vi "energy scan.vi"() -> ()   [LabVIEW 2013]
uses:
  <vilib>/Utility/file.llb/Write To Spreadsheet File (I64).vi
panel:
  in  "encoder enable":bool
  in  "2nd motor enable":bool=TRUE
  out "status":string="motion complete"
  in  "filename":string="cu_foil_Kalpha_01.txt"
  in  "file path":path=path "C:/Users/seidler/Documents/lab XANES software/lab XES data/Joe/Si_111_2013_12_09"
  out "step number":i32=399
  out "detector encoder":string="-189735\r"
  out "source encoder":string="-151316\r"
  in  "detector motor":u16(ring)=5 items=["theta"=1, "chi"=2, "rho"=3, "source"=4, "detector"=5, "sample"=6]
  in  "source motor":u16(ring)=4 items=["theta"=1, "chi"=2, "rho"=3, "source"=4, "detector"=5, "sample"=6]
  out "XY Graph":cluster{i32[], i32[]}(graph)={[0, 1, 2, 3, 4, 5, 6, 7, 8, 9, 10, 11, 12, 13, 14, 15, 16, 17, 18, 19, 20, 21, 22, 23, 24, 25, 26, 27, 28, 29, 30, 31, 32, 33, 34, 35, 36, 37, 38, 39, 40, 41, 42, 43, 44, 45, 46, 47, 48, 49, 50, 51, 52, 53, 54, 55, 56, 57, 58, 59, 60, 61, 62, 63, 64, 65, 66, 67, 68, 69, 70, 71, 72, 73, 74, 75, 76, 77, 78, 79, 80, 81, 82, 83, 84, 85, 86, 87, 88, 89, 90, 91, 92, 93, 94, 95, 96, 97, 98, 99, 100, 101, 102, 103, 104, 105, 106, 107, 108, 109, 110, 111, 112, 113, 114, 115, 116, 117, 118, 119, 120, 121, 122, 123, 124, 125, 126, 127, 128, 129, 130, 131, 132, 133, 134, 135, 136, 137, 138, 139, 140, 141, 142, 143, 144, 145, 146, 147, 148, 149, 150, 151, 152, 153, 154, 155, 156, 157, 158, 159, 160, 161, 162, 163, 164, 165, 166, 167, 168, 169, 170, 171, 172, 173, 174, 175, 176, 177, 178, 179, 180, 181, 182, 183, 184, 185, 186, 187, 188, 189, 190, 191, 192, 193, 194, 195, 196, 197, 198, 199, 200, 201, 202, 203, 204, 205, 206, 207, 208, 209, 210, 211, 212, 213, 214, 215, 216, 217, 218, 219, 220, 221, 222, 223, 224, 225, 226, 227, 228, 229, 230, 231, 232, 233, 234, 235, 236, 237, 238, 239, 240, 241, 242, 243, 244, 245, 246, 247, 248, 249, 250, 251, 252, 253, 254, 255, 256, 257, 258, 259, 260, 261, 262, 263, 264, 265, 266, 267, 268, 269, 270, 271, 272, 273, 274, 275, 276, 277, 278, 279, 280, 281, 282, 283, 284, 285, 286, 287, 288, 289, 290, 291, 292, 293, 294, 295, 296, 297, 298, 299, 300, 301, 302, 303, 304, 305, 306, 307, 308, 309, 310, 311, 312, 313, 314, 315, 316, 317, 318, 319, 320, 321, 322, 323, 324, 325, 326, 327, 328, 329, 330, 331, 332, 333, 334, 335, 336, 337, 338, 339, 340, 341, 342, 343, 344, 345, 346, 347, 348, 349, 350, 351, 352, 353, 354, 355, 356, 357, 358, 359, 360, 361, 362, 363, 364, 365, 366, 367, 368, 369, 370, 371, 372, 373, 374, 375, 376, 377, 378, 379, 380, 381, 382, 383, 384, 385, 386, 387, 388, 389, 390, 391, 392, 393, 394, 395, 396, 397, 398, 399], [20, 23, 14, 17, 19, 21, 27, 19, 23, 16, 20, 22, 21, 26, 21, 24, 21, 18, 21, 19, 27, 23, 25, 22, 24, 16, 18, 25, 21, 25, 23, 25, 27, 19, 22, 24, 33, 27, 26, 34, 32, 24, 23, 26, 35, 29, 31, 28, 35, 30, 26, 41, 38, 38, 30, 30, 36, 47, 43, 44, 45, 42, 48, 49, 47, 49, 31, 53, 49, 50, 52, 51, 57, 66, 63, 64, 68, 75, 68, 89, 74, 64, 104, 113, 94, 106, 98, 158, 133, 141, 186, 184, 192, 200, 225, 279, 242, 314, 312, 398, 411, 502, 542, 520, 736, 787, 859, 960, 1045, 1179, 1285, 1496, 1544, 1613, 1606, 1665, 1557, 1592, 1469, 1286, 1135, 1030, 895, 831, 689, 643, 516, 428, 422, 349, 296, 271, 241, 229, 211, 211, 147, 172, 154, 140, 158, 137, 126, 117, 129, 112, 104, 122, 113, 112, 92, 79, 103, 83, 81, 100, 110, 97, 101, 103, 101, 84, 85, 119, 114, 121, 136, 139, 153, 159, 163, 158, 167, 186, 225, 202, 228, 236, 267, 293, 311, 352, 408, 472, 504, 589, 643, 722, 784, 911, 978, 1183, 1299, 1571, 1750, 2049, 2227, 2431, 2892, 3020, 3211, 3089, 3132, 3048, 2655, 2402, 2016, 1808, 1581, 1335, 1056, 877, 736, 607, 591, 492, 403, 363, 344, 264, 239, 269, 221, 218, 184, 173, 149, 143, 133, 124, 115, 107, 105, 94, 80, 84, 74, 78, 72, 64, 63, 56, 51, 42, 56, 48, 42, 45, 45, 42, 43, 41, 43, 34, 36, 40, 44, 31, 35, 37, 27, 24, 29, 16, 26, 27, 22, 27, 29, 32, 25, 21, 17, 21, 21, 18, 16, 11, 20, 18, 18, 25, 15, 16, 11, 13, 19, 16, 16, 13, 12, 10, 6, 9, 10, 15, 15, 5, 15, 13, 8, 15, 13, 11, 8, 11, 4, 10, 10, 11, 8, 14, 12, 9, 11, 5, 11, 14, 11, 11, 10, 16, 12, 11, 9, 8, 11, 12, 6, 9, 16, 10, 5, 6, 9, 6, 6, 11, 4, 8, 13, 13, 5, 15, 8, 6, 8, 5, 4, 5, 14, 5, 9, 1, 9, 11, 5, 10, 5, 11, 8, 10, 7, 6, 8, 5, 5, 7, 7, 6, 4, 4, 9, 3, 3, 3, 4, 7, 8, 3, 4, 3, 3, 4, 3, 2, 6, 4, 7, 3, 3, 2, 3, 2, 3, 2, 5, 6, 7, 4]}
  out "Waveform Chart":i32(graph)=4
  in  "number of steps":i16=400
  in  "step size":i16=1000
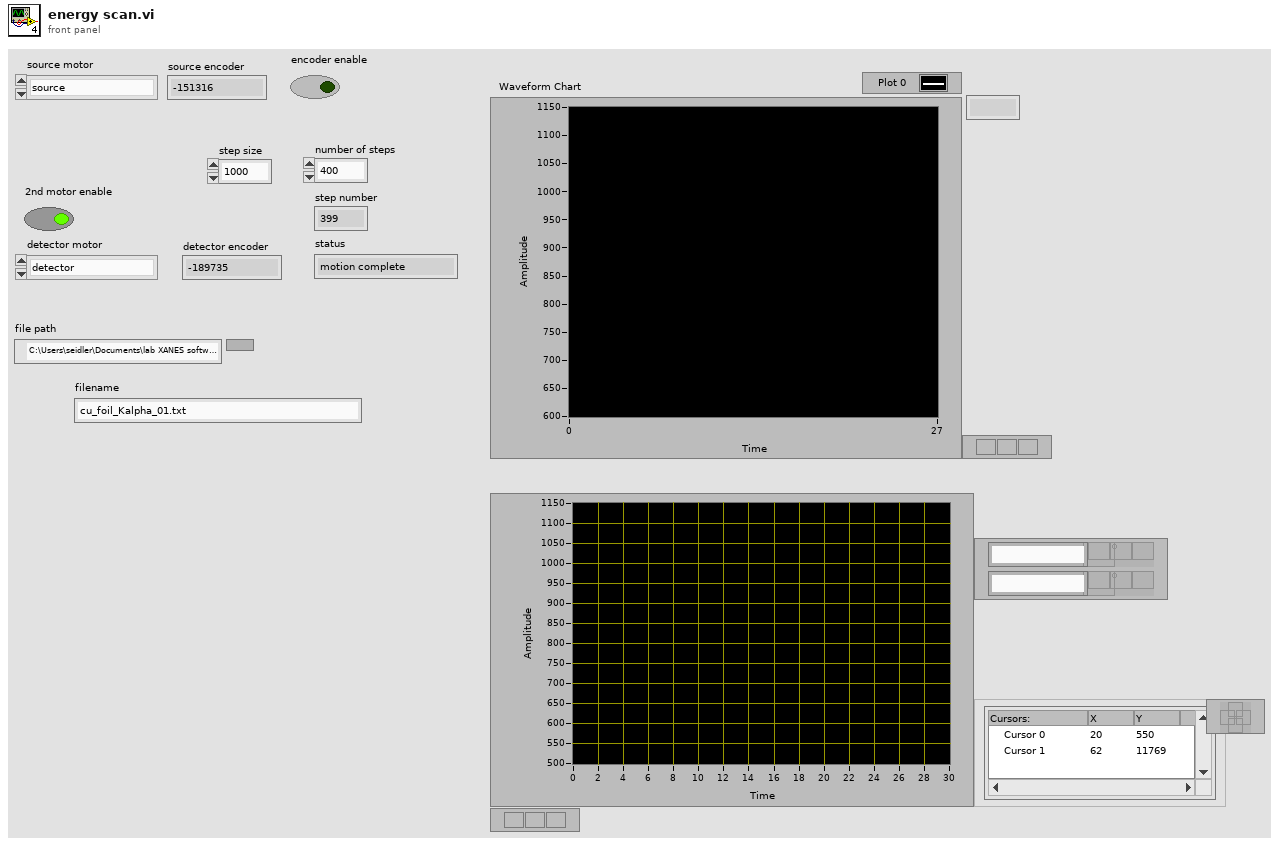
[diagram p1: front panel]
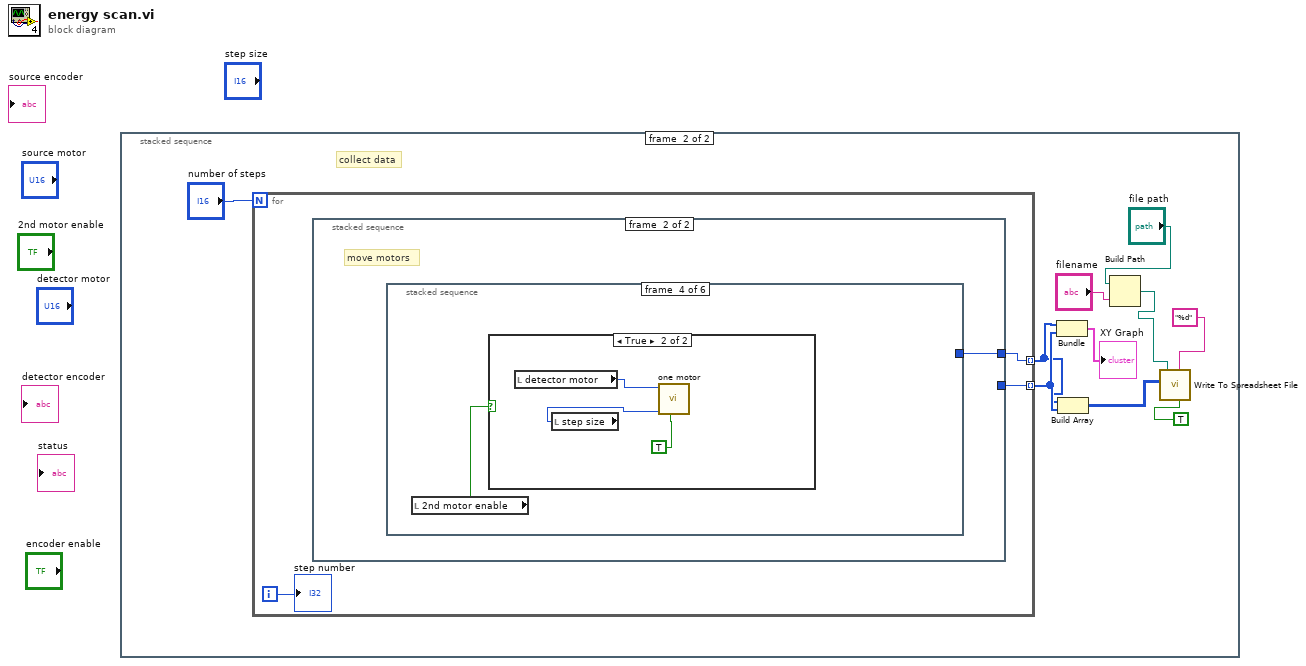
[diagram p0: block diagram]
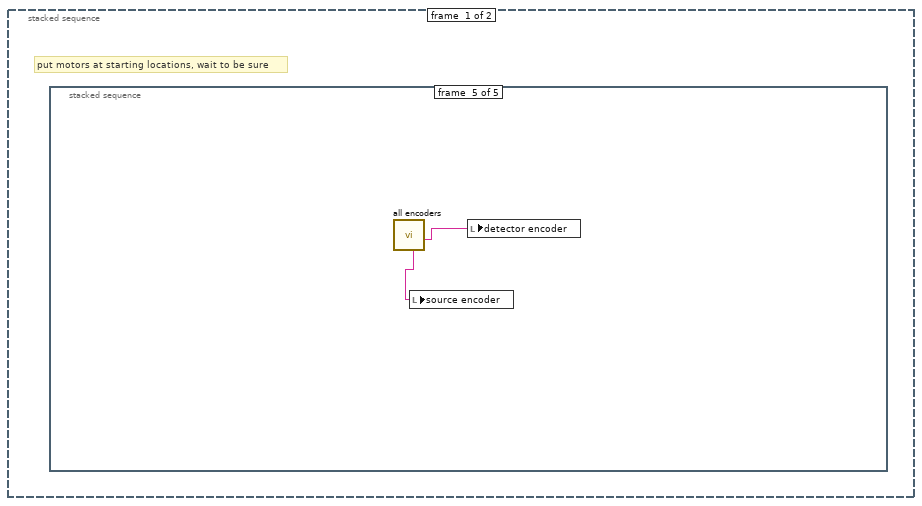
[diagram p2: hidden frame]
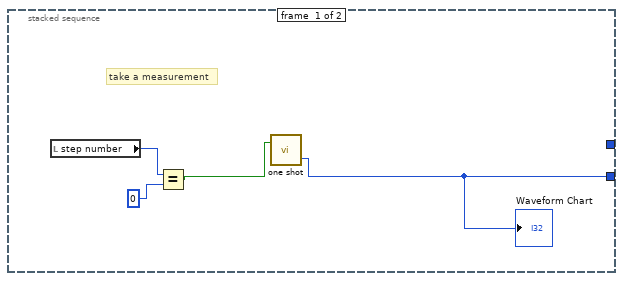
[diagram p7: hidden frame]
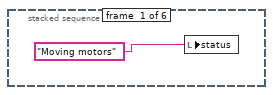
[diagram p8: hidden frame]
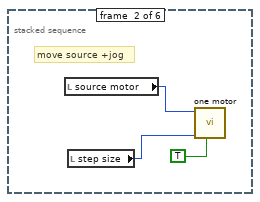
[diagram p9: hidden frame]
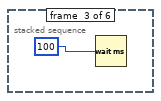
[diagram p10: hidden frame]
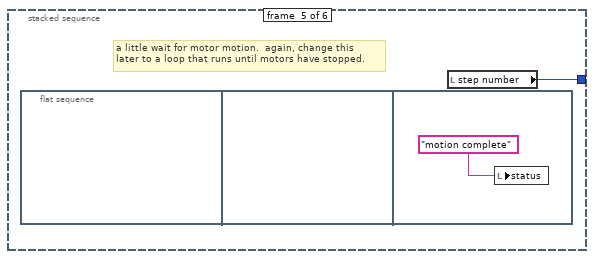
[diagram p12: hidden frame]
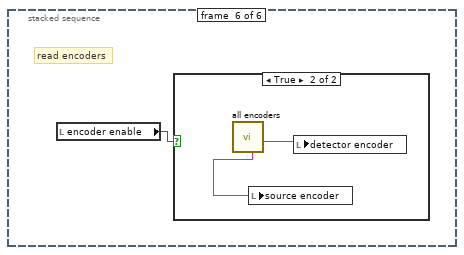
[diagram p13: hidden frame]
diagram:
  n1 = stacked-sequence {
    frame #0 {
      # "put motors at starting locations, wait to be sure"
      n2 = stacked-sequence {
        frame #0 {
        }
        frame #1 {
        }
        frame #2 {
        }
        frame #3 {
          # "10sec wait for motor move.  \nchange this later to a loop that checks to see that motors have halted."
        }
        frame #4 {
          n3 = call "all encoders.vi"() -> ("source encoder"=w1:string, "detector encoder"=w2:string)  [unwired: 1 in, 4 out]
          n4 = local write "source encoder"(w1) -> ()
          n5 = local write "detector encoder"(w2) -> ()
        }
      }
    }
    frame #1 {
      # "collect data"
      n6 = for {
        N: "number of steps" -> [_]
        tunnel: [w15] -> w10 mode=indexing
        tunnel: [w13] -> w9 mode=indexing
        i -> [w14]
        n7 = stacked-sequence {
          tunnel: [w19 _] -> w15
          tunnel: [_ w20] -> w13
          frame #0 {
            # "take a measurement"
            n8 = local read "step number"() -> (w16:i32)
            n9 = Equal?(x=w16, y=0) -> (x = y?=w17:bool)
            n10 = call "one shot.vi"("first point"=w17) -> ("ROI counts"=w19:i32)  [unwired: 1 in, 1 out]
            "Waveform Chart" <- w19
          }
          frame #1 {
            # "move motors"
            n11 = stacked-sequence {
              tunnel: [_ _ _ _ w30 _] -> w20
              frame #0 {
                n12 = local write "status"("Moving motors") -> ()
              }
              frame #1 {
                # "move source +jog"
                n13 = local read "source motor"() -> (w24:u16)
                n14 = local read "step size"() -> (w23:i16)
                n15 = call "one motor.vi"("Jog plus"=TRUE, "Jog"=w23, "motor name"=w24) -> ()  [unwired: 7 in, 2 out]
              }
              frame #2 {
                n16 = Wait (ms)(milliseconds to wait=100) -> ()  [unwired: 1 out]
              }
              frame #3 {
                n17 = local read "2nd motor enable"() -> (w26:bool)
                n18 = case shown="True" w26 {
                  frame False {
                  }
                  frame True {
                    n19 = local read "detector motor"() -> (w29:u16)
                    n20 = local read "step size"() -> (w28:i16)
                    n21 = call "one motor.vi"("Jog plus"=TRUE, "Jog"=w28, "motor name"=w29) -> ()  [unwired: 7 in, 2 out]
                  }
                }
              }
              frame #4 {
                # "a little wait for motor motion.  again, change this \nlater to a loop that runs until motors have stopped."
                n22 = flat-sequence {
                  frame #0 {
                  }
                  frame #1 {
                  }
                  frame #2 {
                    n23 = local write "status"("motion complete") -> ()
                  }
                }
                n24 = local read "step number"() -> (w30:i32)
              }
              frame #5 {
                # "read encoders"
                n25 = local read "encoder enable"() -> (w32:bool)
                n26 = case shown="True" w32 {
                  frame False {
                  }
                  frame True {
                    n27 = call "all encoders.vi"() -> ("source encoder"=w34:string, "detector encoder"=w33:string)  [unwired: 1 in, 4 out]
                    n28 = local write "source encoder"(w34) -> ()
                    n29 = local write "detector encoder"(w33) -> ()
                  }
                }
              }
            }
          }
        }
        "step number" <- w14
      }
      n30 = Bundle(w9, w10) -> (→"XY Graph":cluster{i32[], i32[]})  [unwired: 1 in]
      n31 = Build Array(w9, w10) -> (w8:i32[][])
      n32 = Build Path(base path="file path", name or relative path="filename") -> (appended path=w3:path)
      n33 = call-poly <vilib>:"Write To Spreadsheet File.vi"("transpose? (no:F)"=TRUE, "format (%d)"="%d", "2D data"=w8, "file path (dialog if empty)"=w3) -> ()  [unwired: 4 in, 1 out]
    }
  }
